vi "Zero.vi"(0 "Power Detector in":refnum<class "Power Detector.lvclass">, 11 "error in":errorcluster) -> (4 "Power Detector out":refnum<class "Power Detector.lvclass">, 15 "error out":errorcluster)   [LabVIEW 2023, in "NI CAL-5501 Power Detector.lvlib" / "Power Detector.lvclass"]
uses:
  Power Detector.lvclass
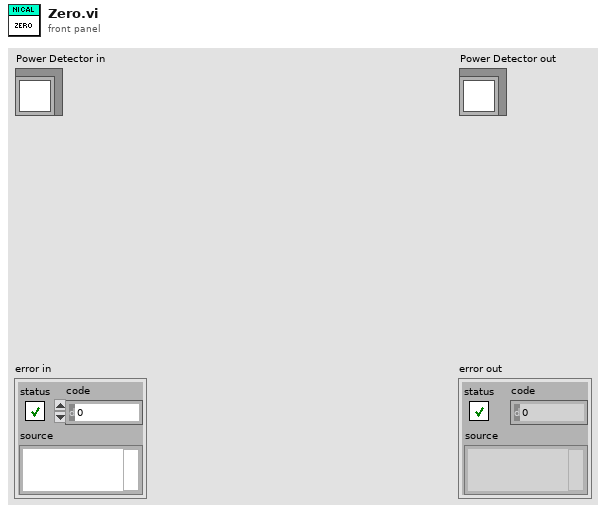
[diagram p1: front panel]
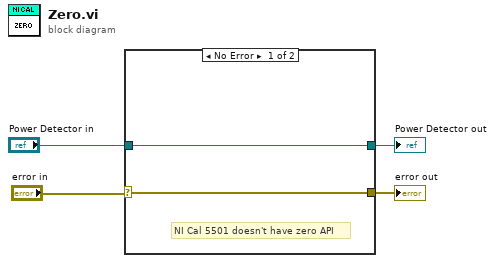
[diagram p0: block diagram]
diagram:
  n1 = case shown="No Error" "error in" {
    selector: "error in" -> [w6 w7]
    tunnel: [w6 w7] -> w3
    tunnel: [w5 w8] -> w2
    tunnel: "Power Detector in" -> [w5 w8]
    frame No Error {
      # "NI Cal 5501 doesn't have zero API"
    }
    frame Error {
    }
  }
  "error out" <- w3
  "Power Detector out" <- w2
